vi "Create Waterfall.vi"(6 "Draw Mode":T8(ring)=enum."Triangles", 7 "3D Waterfall Property":T1={"General Property"={"Plot Name"="", "Coordinate System"=enum."Cartesian", "Opacity"=0.0}, "Projection Property"={"Draw XY"=FALSE, "Draw YZ"=FALSE, "Draw XZ"=FALSE}, "Plot Property"={"Line Style"=enum."None", "Line Width"=0.0, "Color Ramp Cluster"={"Color Ramp Style"=enum."None", "Color Ramp Array"=[16711934, 393471, 57855, 4390754, 16449346, 16744722, 16711680], "Color Ramp Index"=[45, 91, 133, 175, 219, 255], "Interpolate?"=FALSE, "Logarithm?"=FALSE}, "Antialiasing"=FALSE}, "Waterfall Property"={"Waterfall Mode"=enum."Lines"}}, 8 "error in (no error)":errorcluster, 9 "Actual Transform In":T7, 10 "Plot Representation In":T4, 11 "Plot Object In":refnum<vi>) -> (0 "error out":errorcluster, 1 "Actual Transform Out":T7, 2 "Plot Representation Out":T4, 3 "Plot Object Out":refnum<vi>, 4 "Waterfall Object Out":refnum<vi>)   [LabVIEW 2017, in "3D Waterfall.lvclass"]
uses:
  <vilib>/Math Plots/3D Math Plots/3D Waterfall/3D Waterfall/3D Waterfall.lvclass
  <vilib>/Math Plots/3D Math Plots/3D Plot/3D Plot/Typedef/Actual Transform.ctl
  <vilib>/Math Plots/3D Math Plots/3D Plot/3D Plot/Typedef/Range Clusters.ctl
  <vilib>/Math Plots/3D Math Plots/3D Plot/3D Plot/Typedef/Plot Representation.ctl
  <vilib>/Math Plots/3D Math Plots/3D Plot/3D Plot/Typedef/Mesh Data.ctl
  <vilib>/Math Plots/3D Math Plots/3D Waterfall/3D Waterfall/Typedef/3D Waterfall Property.ctl
  <vilib>/Math Plots/3D Math Plots/3D Plot/3D Plot/Typedef/Line Type.ctl
  <vilib>/Math Plots/3D Math Plots/3D Plot/3D Plot/Typedef/Color Ramp Cluster.ctl
  <vilib>/picture/3D Picture Control/NI_3D Picture Control.lvlib
  <vilib>/Math Plots/3D Math Plots/3D Plot/3D Plot/3D Plot.lvclass
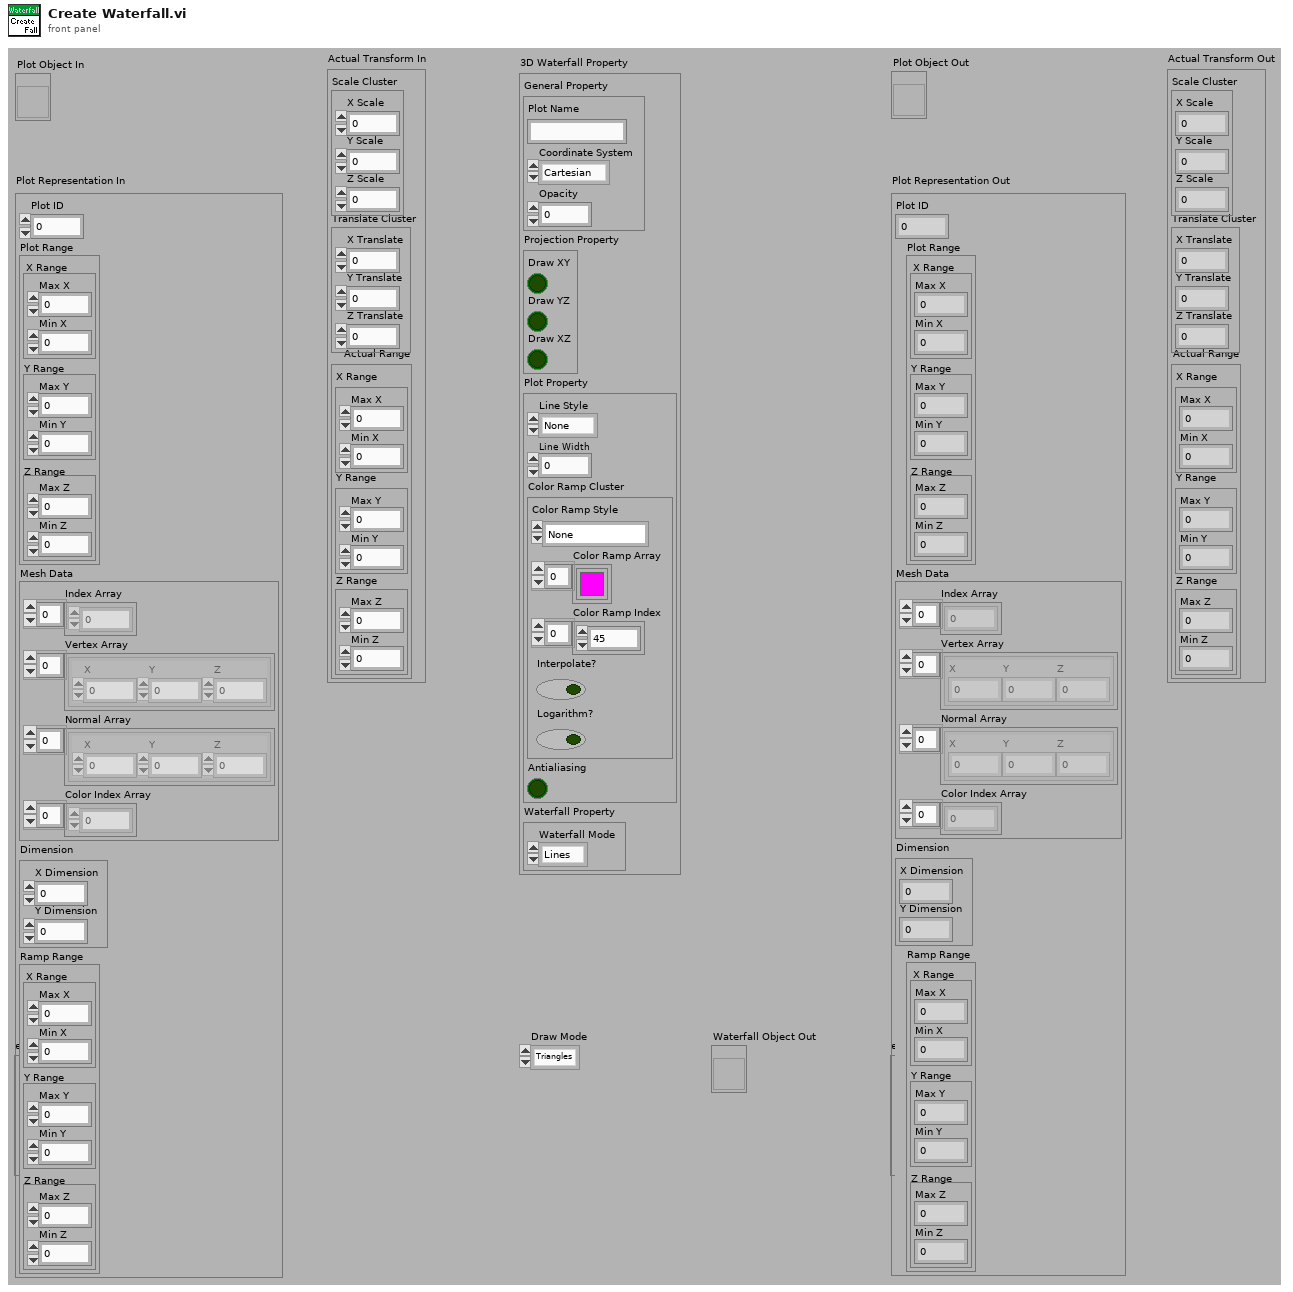
[diagram p1: front panel]
types:
  T1 = typedef "3D Waterfall.lvclass/3D Waterfall Property.ctl" = cluster{"General Property":cluster{"Plot Name":string, "Coordinate System":enum16{"Cartesian", "Cylindrical", "Spherical"}, "Opacity":sgl}, "Projection Property":cluster{"Draw XY":bool, "Draw YZ":bool, "Draw XZ":bool}, "Plot Property":cluster{"Line Style":T2, "Line Width":sgl, "Color Ramp Cluster":T3, "Antialiasing":bool}, "Waterfall Property":cluster{"Waterfall Mode":enum16{"Lines", "Slices"}}}
  T2 = typedef "3D Plot.lvclass/Line Type.ctl" = enum16{"None", "Solid", "Dash", "Dot", "Dash Dot"}
  T3 = typedef "3D Plot.lvclass/Color Ramp Cluster.ctl" = cluster{"Color Ramp Style":enum16{"None", "Shaded", "Color spectrum", "Grey scale", "Custom"}, "Color Ramp Array":u32[], "Color Ramp Index":i32[], "Interpolate?":bool, "Logarithm?":bool}
  T4 = typedef "3D Plot.lvclass/Plot Representation.ctl" = cluster{"Plot ID":i32, "Plot Range":T5, "Mesh Data":T6, "Dimension":cluster{"X Dimension":i32, "Y Dimension":i32}, "Ramp Range":T5}
  T5 = typedef "3D Plot.lvclass/Range Clusters.ctl" = cluster{"X Range":cluster{"Max X":sgl, "Min X":sgl}, "Y Range":cluster{"Max Y":sgl, "Min Y":sgl}, "Z Range":cluster{"Max Z":sgl, "Min Z":sgl}}
  T6 = typedef "3D Plot.lvclass/Mesh Data.ctl" = cluster{"Index Array":u32[], "Vertex Array":cluster{"X":sgl, "Y":sgl, "Z":sgl}[], "Normal Array":cluster{"X":sgl, "Y":sgl, "Z":sgl}[], "Color Index Array":i32[]}
  T7 = typedef "3D Plot.lvclass/Actual Transform.ctl" = cluster{"Scale Cluster":cluster{"X Scale":sgl, "Y Scale":sgl, "Z Scale":sgl}, "Translate Cluster":cluster{"X Translate":sgl, "Y Translate":sgl, "Z Translate":sgl}, "Actual Range":T5}
  T8 = enum16{"Points", "Lines", "Line Strip", "Line Loop", "Triangles", "Triangle Strip", "Triangle Fan", "Quads", "Quad Strip", "Polygon"}
  T9 = enum16{"Overall", "Per Primitive", "Per Vertex", "Binding Off"}
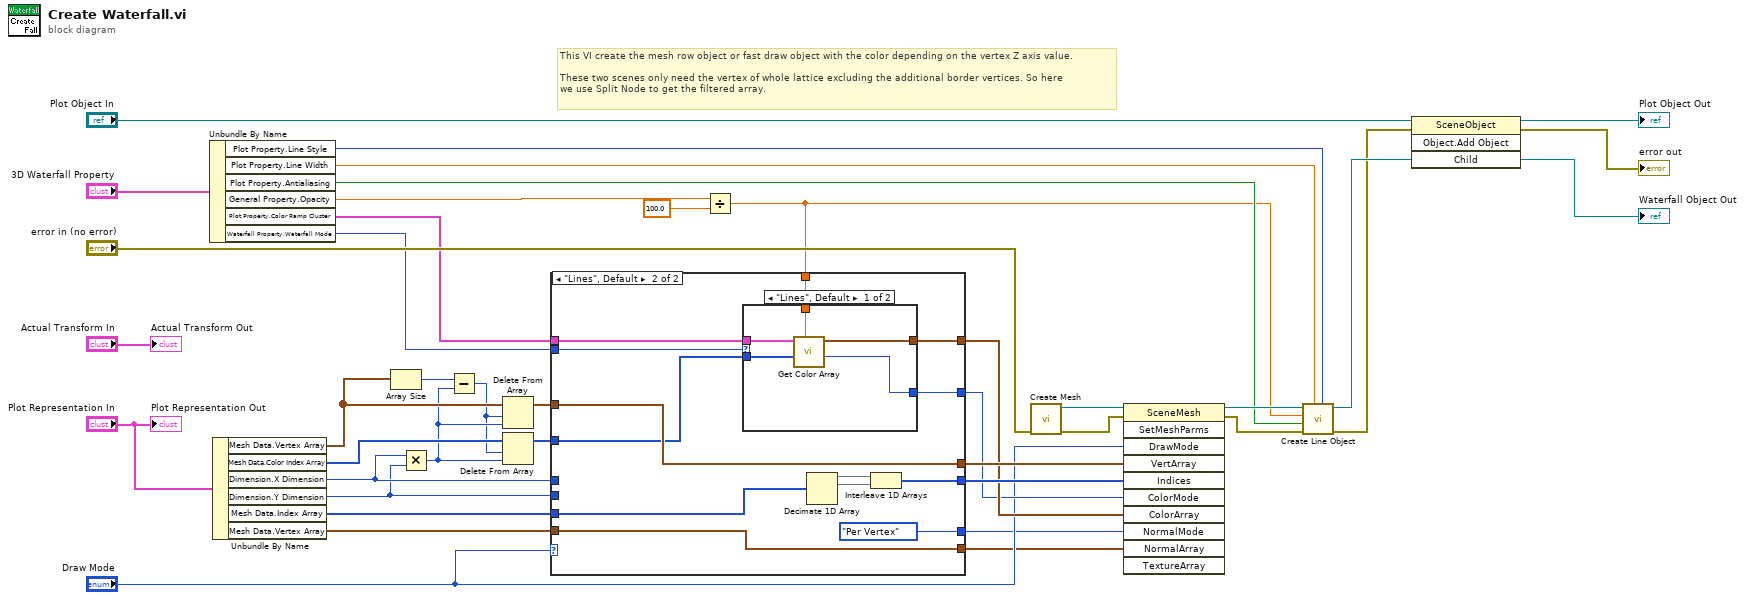
[diagram p0: block diagram]
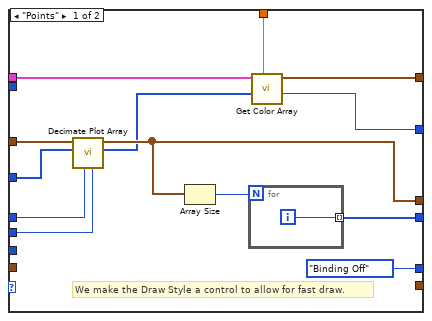
[diagram p2: hidden frame]
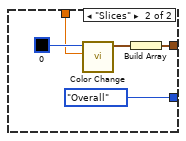
[diagram p3: hidden frame]
diagram:
  # "This VI create the mesh row object or fast draw object with the color depending on the vertex Z axis value.\n\nThese two scenes only need the vertex of whole lattice excluding the additional border vertices. So here\nwe use Split Node to get the filtered array."
  n1 = Unbundle By Name("3D Waterfall Property") -> ("Plot Property.Line Style"=w15:T2, "Plot Property.Line Width"=w16:sgl, "Plot Property.Antialiasing"=w13:bool, "General Property.Opacity"=w14:sgl, "Plot Property.Color Ramp Cluster"=w28:T3, "Waterfall Property.Waterfall Mode"=w10:enum16{"Lines", "Slices"})
  n2 = Unbundle By Name("Plot Representation In") -> ("Mesh Data.Vertex Array"=w5:cluster{"X":sgl, "Y":sgl, "Z":sgl}[], "Mesh Data.Color Index Array"=w6:i32[], "Dimension.X Dimension"=w23:i32, "Dimension.Y Dimension"=w22:i32, "Mesh Data.Index Array"=w8:u32[], "Mesh Data.Vertex Array"=w9:cluster{"X":sgl, "Y":sgl, "Z":sgl}[])
  n3 = Array Size(array=w5) -> (size(s)=w7:i32)
  n4 = Multiply(x=w23, y=w22) -> (x*y=w3:i32)
  n5 = Subtract(x=w7, y=w3) -> (x-y=w2:i32)
  n6 = Delete From Array(array=w5, length=w2, index=w3) -> (array with subset deleted=w4:cluster{"X":sgl, "Y":sgl, "Z":sgl}[])  [unwired: 1 out]
  n7 = Delete From Array(array=w6, length=w2, index=w3) -> (array with subset deleted=w1:i32[])  [unwired: 1 out]
  n8 = Divide(x=w14, y=sgl 100.0) -> (x/y=w12:sgl)
  n9 = case shown="\"Lines\", Default" "Draw Mode" {
    tunnel: w4 -> [w52 w64]
    tunnel: [w49 w64] -> w30
    tunnel: w8 -> [_ w59]
    tunnel: [w44 w58] -> w32
    tunnel: w9 -> [_ w65]
    tunnel: [_ w65] -> w24
    tunnel: w23 -> [w51 _]
    tunnel: w22 -> [w50 _]
    tunnel: w28 -> [w43 w57]
    tunnel: w12 -> [w46 w62]
    tunnel: [w48 w67] -> w27
    tunnel: [w47 w66] -> w26
    tunnel: w1 -> [w45 w63]
    tunnel: [T9."Binding Off" ("Normal Binding Mode") T9."Per Vertex" ("Normal Binding Mode")] -> w11
    tunnel: w10 -> [_ w55]
    frame "Points" {
      # "We make the Draw Style a control to allow for fast draw."
      n10 = call <vilib>:"Decimate Plot Array.vi"("Y Dimension"=w50, "X Dimension"=w51, "Color Index Array In"=w45, "Vertex Array In"=w52) -> ("Color Index Array Out"=w41:i32[], "Vertex Array Out"=w49:cluster{"X":sgl, "Y":sgl, "Z":sgl}[])  [unwired: 1 in, 5 out]
      n11 = Array Size(array=w49) -> (size(s)=w53:i32)
      n12 = for {
        N: w53 -> [_]
        tunnel: [w54] -> w44 mode=indexing
        i -> [w54]
      }
      n13 = call <vilib>:"Get Color Array.vi"("Alpha"=w46, "Color Index Array"=w41, "Color Ramp Cluster"=w43) -> ("Color Binding Mode"=w47:T9, "Color Array"=w48:cluster{"R":sgl, "G":sgl, "B":sgl, "A":sgl}[])  [unwired: 4 in, 3 out]
    }
    frame "Lines", Default {
      n14 = case shown="\"Lines\", Default" w55 {
        tunnel: [w72 w76] -> w67
        tunnel: [w71 T9."Overall" ("Color Binding Mode")] -> w66
        tunnel: w63 -> [w70 _]
        tunnel: w62 -> [w69 w73]
        tunnel: w57 -> [w68 _]
        frame "Lines", Default {
          n15 = call <vilib>:"Get Color Array.vi"("Alpha"=w69, "Color Index Array"=w70, "Color Ramp Cluster"=w68) -> ("Color Binding Mode"=w71:T9, "Color Array"=w72:cluster{"R":sgl, "G":sgl, "B":sgl, "A":sgl}[])  [unwired: 4 in, 3 out]
        }
        frame "Slices" {
          n16 = call <vilib>:"Color Change.vi"("Alpha"=w73, "Color"=u32 0) -> ("RGBA"=w77:cluster{"R":sgl, "G":sgl, "B":sgl, "A":sgl})  [unwired: 9 out]
          n17 = Build Array(w77) -> (w76:cluster{"R":sgl, "G":sgl, "B":sgl, "A":sgl}[])
        }
      }
      n18 = Decimate 1D Array(w59) -> (w61:u32[], w60:u32[])  [unwired: 2 out]
      n19 = Interleave 1D Arrays(w61, w60) -> (w58:u32[])
    }
  }
  n20 = call <vilib>:"Create Mesh.vi"("error in (no error)"="error in (no error)") -> ("error out"=w31:errorcluster, "New Mesh Refnum"=w33:refnum<vi>)  [unwired: 9 out]
  n21 = invoke class="SceneMesh" method="SetMeshParms"(reference=w33, error in=w31, "DrawMode"="Draw Mode", "VertArray"=w30, "Indices"=w32, "ColorMode"=w26, "ColorArray"=w27, "NormalMode"=w11, "NormalArray"=w24) -> (reference out=w18:refnum<vi>, error out=w17:errorcluster)  [unwired: 2 in, 9 out]
  n22 = call <vilib>:"Create Line Object.vi"("Line Style"=w15, "Line Width"=w16, "error in (no error)"=w17, "Antialiasing"=w13, "Alpha"=w12, "Mesh Ref In"=w18) -> ("error out"=w19:errorcluster, "Object Ref Out"=w20:refnum<vi>)  [unwired: 4 out]
  n23 = invoke class="SceneObject" method="Object.Add Object"(reference="Plot Object In", error in=w19, "Child"=w20) -> (reference out=→"Plot Object Out":refnum<vi>, error out=→"error out":errorcluster, "Child"=→"Waterfall Object Out":refnum<vi>)  [unwired: 1 in, 1 out]
  "Actual Transform Out" <- "Actual Transform In"
  "Plot Representation Out" <- "Plot Representation In"
